vi "Bar100GetCalibration.vi"() -> ()   [LabVIEW 2019]
uses:
  <vilib>/myRIO/Instrument Drivers/Onboard IO/I2C/I2C.lvlib
  <vilib>/myRIO/Instrument Drivers/Onboard IO/I2C/typedefs/I2C Transfer Rate.ctl
  <vilib>/myRIO/Instrument Drivers/Onboard IO/I2C/typedefs/I2C Configuration.ctl
  <vilib>/myRIO/Common/Instrument Driver Framework/myRIO v1.0/I2C/typedefs/I2C Channels Enum.ctl
  <vilib>/myRIO/Common/Instrument Driver Framework/Utilities/typedefs/Generic FPGA Reference.ctl
  <vilib>/myRIO/Common/Instrument Driver Framework/Utilities/typedefs/myRIO v1.0 Reference.ctl
  <vilib>/myRIO/Common/Instrument Driver Framework/Utilities/typedefs/Hardware Version Enum.ctl
  <vilib>/myRIO/Common/Instrument Driver Framework/Utilities/typedefs/myRIO Generic Hardware Reference.ctl
  <vilib>/myRIO/Instrument Drivers/Onboard IO/I2C/typedefs/I2C Reference.ctl
  <vilib>/myRIO/Instrument Drivers/Onboard IO/I2C/vis/myRIO I2C Open.xnode
  <vilib>/myRIO/Common/Instrument Driver Framework/myRIO v1.0/I2C/vis/myRIO v1.1 Open I2C.vi
  <vilib>/userDefined/High Color/nirio_resource_hc.ctl
  <vilib>/myRIO/Instrument Drivers/Onboard IO/I2C/typedefs/I2C User Configuration.ctl
panel:
  out "mode":u32
  out "P_mode":dbl
  out "P_max":dbl
  out "P_min":dbl
  out "error out":errorcluster
  in  "error in (no error)":errorcluster
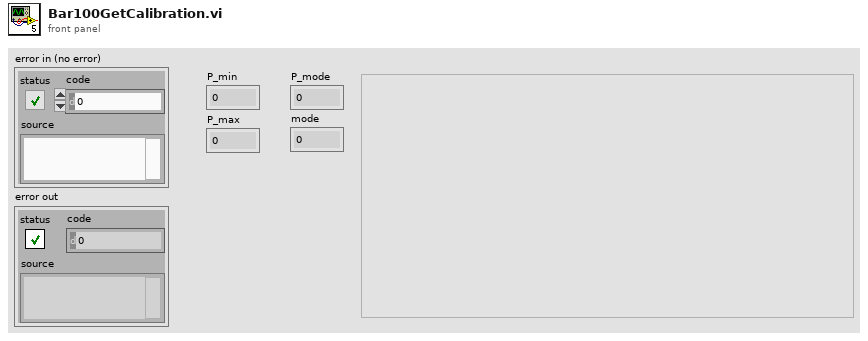
[diagram p1: front panel]
types:
  T1 = typedef "I2C.lvlib/I2C User Configuration.ctl" = cluster{"I2C Transfer Rate":T2}
  T2 = typedef "I2C.lvlib/I2C Transfer Rate.ctl" = enum16{"Standard mode (100 kbps)", "Fast mode (400 kbps)"}
  T3 = typedef "I2C.lvlib/I2C Reference.ctl" = cluster{"myRIO Reference":T4, "I2C Channels Enum":T8, "I2C Configuration":T9}
  T4 = typedef "myRIO Generic Hardware Reference.ctl" = cluster{"myRIO Model":T5, "myRIO Hardware Reference":T6}
  T5 = typedef "Hardware Version Enum.ctl" = enum16{"Unknown", "myRIO-1900", "myRIO-1950", "roboRIO", "NI ELVIS RIO CM", "ELVIS III"}
  T6 = typedef "myRIO v1.0 Reference.ctl" = cluster{"Generic FPGA Reference":T7, "Allow multiple opens":bool}
  T7 = typedef "Generic FPGA Reference.ctl" = refnum<k20>
  T8 = typedef "I2C Channels Enum.ctl" = enum16{"Not Connected", "A/I2C", "B/I2C", "I2C/I2C"}
  T9 = typedef "I2C.lvlib/I2C Configuration.ctl" = cluster{"I2C Transfer Rate":T2}
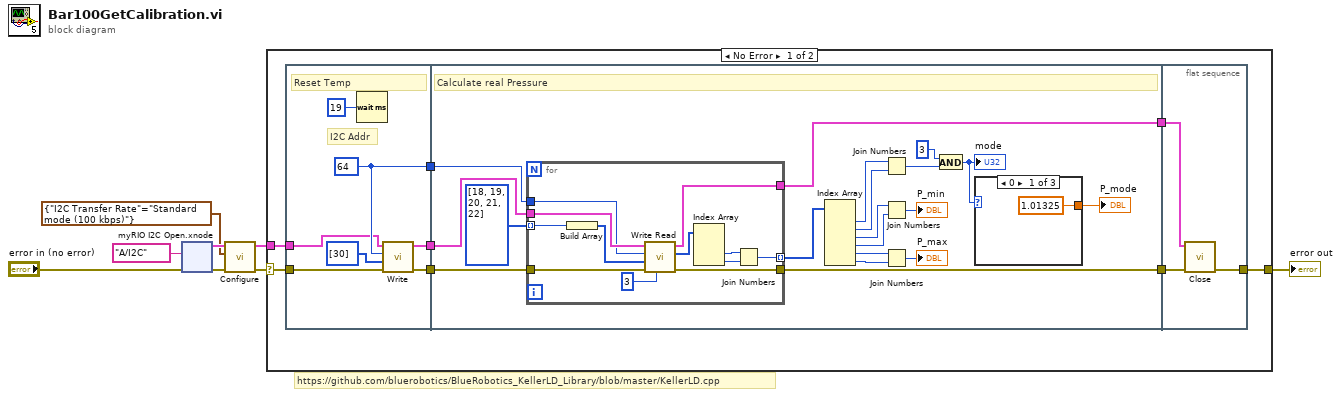
[diagram p0: block diagram]
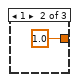
[diagram p2: hidden frame]
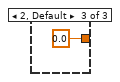
[diagram p3: hidden frame]
diagram:
  # "https://github.com/bluerobotics/BlueRobotics_KellerLD_Library/blob/master/KellerLD.cpp"
  n1 = xnode "myRIO I2C Open.xnode"("error in (no error)"="error in (no error)", "Channel Name"=tag "A/I2C") -> ("error out"=w6:errorcluster, "I2C Ref Out"=w5:T3)  [unwired: 1 in]
  n2 = call <vilib>:"Configure.vi"("error in (no error)"=w6, "I2C User Configuration"=T1 {"I2C Transfer Rate"=enum."Standard mode (100 kbps)"}, "I2C Ref In"=w5) -> ("error out"=w7:errorcluster, "I2C Ref Out"=w8:T3)  [unwired: 7 in]
  n3 = case shown="No Error" w7 {
    selector: w7 -> [w12 w61]
    tunnel: w8 -> [w13 _]
    tunnel: [w9 w61] -> w1
    frame No Error {
      n4 = flat-sequence {
        tunnel: [w23] -> w16
        tunnel: [w22] -> w15
        tunnel: [w21] -> w14
        tunnel: w12 -> [w19]
        tunnel: w13 -> [w18]
        tunnel: w14 -> [w41]
        tunnel: w15 -> [w42]
        tunnel: w16 -> [w39]
        tunnel: [w38] -> w11
        tunnel: [w37] -> w10
        tunnel: w11 -> [w60]
        tunnel: w10 -> [w59]
        tunnel: [w58] -> w9
        frame #0 {
          w23 = u8 64 ("Slave Address (7-bit)")
          # "I2C Addr"
          # "Reset Temp"
          n5 = Wait (ms)(milliseconds to wait=u32 19) -> ()  [unwired: 1 out]
          n6 = call <vilib>:"Write.vi"("error in (no error)"=w19, "Bytes to Write"=u8[] [30], "Slave Address (7-bit)"=w23, "I2C Ref In"=w18) -> ("error out"=w21:errorcluster, "I2C Ref Out"=w22:T3)  [unwired: 6 in]
        }
        frame #1 {
          # "Calculate real Pressure"
          n7 = for {
            tunnel: w42 -> [w57]
            tunnel: w41 -> [w56]
            tunnel: u8[] [18, 19, 20, 21, 22] ("Bytes to Write") -> [w53] mode=indexing
            tunnel: w39 -> [w54]
            tunnel: [w51] -> w38
            tunnel: [w50] -> w37
            tunnel: [w46] -> w36 mode=indexing
            n8 = Build Array(w53) -> (w52:u8[])
            n9 = call <vilib>:"Write Read.vi"("Byte Count"=u32 3, "error in (no error)"=w56, "Bytes to Write"=w52, "Slave Address (7-bit)"=w54, "I2C Ref In"=w57) -> ("error out"=w50:errorcluster, "Bytes Read"=w49:u8[], "I2C Ref Out"=w51:T3)  [unwired: 3 in]
            n10 = Index Array(array=w49) -> (element #2=w48:u8, element #3=w47:u8)  [unwired: 3 in, 1 out]
            n11 = Join Numbers(hi=w48, lo=w47) -> ((hi.lo)=w46:u16)
          }
          n12 = Index Array(array=w36) -> (element #1=w29:u16, element #2=w28:u16, element #3=w35:u16, element #4=w34:u16, element #5=w33:u16, element #6=w32:u16)  [unwired: 6 in]
          n13 = Join Numbers(hi=w29, lo=w28) -> ((hi.lo)=w27:u32)
          n14 = Join Numbers(hi=w35, lo=w34) -> ((hi.lo)=→"P_min":u32)
          n15 = Join Numbers(hi=w33, lo=w32) -> ((hi.lo)=→"P_max":u32)
          n16 = And(x=u32 3, y=w27) -> (x .and. y?=w25:u32)
          "mode" <- w25
          n17 = case shown="0" w25 {
            tunnel: [1.01325 1.0 0.0] -> w24
            frame 0 {
            }
            frame 1 {
            }
            frame 2, Default {
            }
          }
          "P_mode" <- w24
        }
        frame #2 {
          n18 = call <vilib>:"Close.vi"("error in (no error)"=w59, "I2C Ref In"=w60) -> ("error out"=w58:errorcluster)  [unwired: 9 in]
        }
      }
    }
    frame Error {
    }
  }
  "error out" <- w1
